vi "Calculate Label Position.vi"(6 "scaling factor":T3={"horizontal"=1.0, "vertical"=1.0} {"vertical" min=0.0; "horizontal" min=0.0}, 8 "layout owner bounds":T4, 9 "scaled object size":T1, 10 "layout object size":T1, 11 "layout label position":T2) -> (3 "scaled label position":T2)   [LabVIEW 2010, in "NI_SE_Front Panel Layout.lvlib"]
uses:
  NI_SE_Front Panel Layout.lvlib
  <vilib>/Utility/miscctls.llb/LVRectTypeDef.ctl
  <vilib>/Utility/miscctls.llb/LVPositionTypeDef.ctl
  XY Scaling Factor.ctl
  <vilib>/Utility/miscctls.llb/LVBoundsTypeDef.ctl
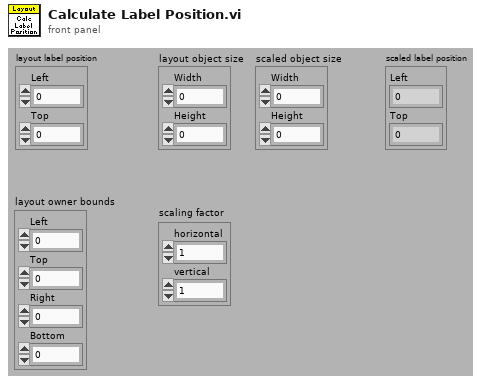
[diagram p1: front panel]
types:
  T1 = typedef "LVBoundsTypeDef.ctl" = cluster{"Width":u32, "Height":u32}
  T2 = typedef "LVPositionTypeDef.ctl" = cluster{"Left":i32, "Top":i32}
  T3 = typedef "NI_SE_Front Panel Layout.lvlib/XY Scaling Factor.ctl" = cluster{"horizontal":dbl, "vertical":dbl}
  T4 = typedef "LVRectTypeDef.ctl" = cluster{"Left":i16, "Top":i16, "Right":i16, "Bottom":i16}
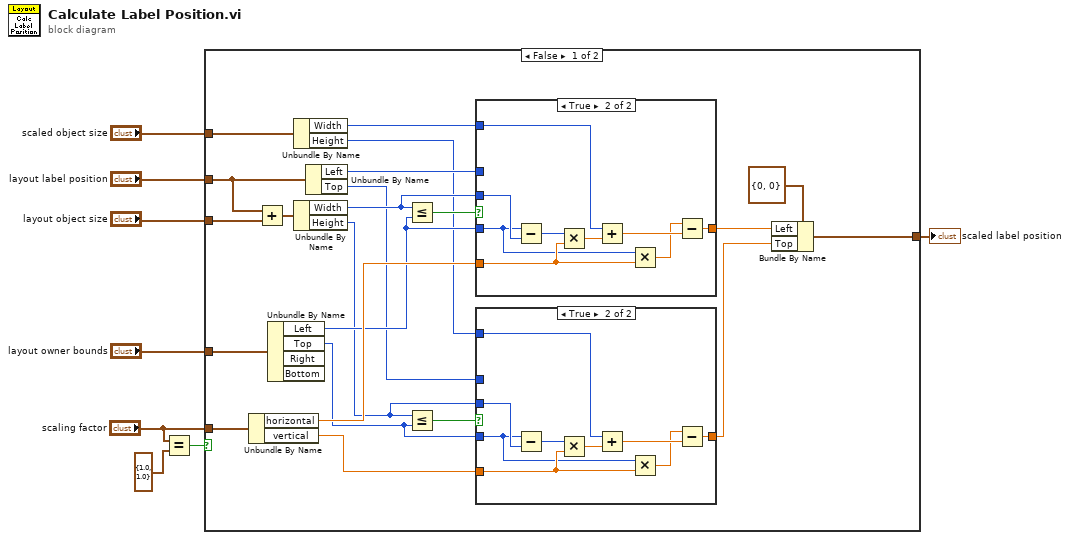
[diagram p0: block diagram]
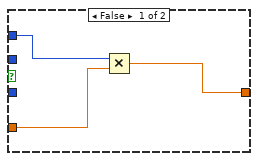
[diagram p2: hidden frame]
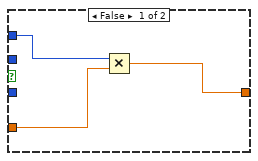
[diagram p3: hidden frame]
diagram:
  n1 = Equal?(x="scaling factor", y=T3 {"horizontal"=1.0, "vertical"=1.0}) -> (x = y?=w2:bool)
  n2 = case shown="False" w2 {
    tunnel: "layout owner bounds" -> [w30 _]
    tunnel: [w27 w55] -> w7
    tunnel: "layout object size" -> [w19 _]
    tunnel: "layout label position" -> [w17 w55]
    tunnel: "scaling factor" -> [w22 _]
    tunnel: "scaled object size" -> [w21 _]
    frame False {
      n3 = Unbundle By Name(w22) -> ("horizontal"=w24:dbl, "vertical"=w13:dbl)
      n4 = Add(x=w17, y=w19) -> (x+y=w18:T1)
      n5 = Unbundle By Name(w30) -> ("Left"=w23:i16, "Top"=w10:i16)  [unwired: 2 out]
      n6 = Unbundle By Name(w21) -> ("Width"=w20:u32, "Height"=w15:u32)
      n7 = Unbundle By Name(w18) -> ("Width"=w25:u32, "Height"=w11:u32)
      n8 = Unbundle By Name(w17) -> ("Left"=w16:i32, "Top"=w14:i32)
      n9 = Less Or Equal?(x=w25, y=w23) -> (x <= y?=w26:bool)
      n10 = Less Or Equal?(x=w11, y=w10) -> (x <= y?=w12:bool)
      n11 = case shown="True" w26 {
        tunnel: [w43 w46] -> w28
        tunnel: w25 -> [_ w54]
        tunnel: w24 -> [w44 w50]
        tunnel: w23 -> [_ w49]
        tunnel: w20 -> [_ w51]
        tunnel: w16 -> [w45 _]
        frame False {
          n12 = Multiply(x=w45, y=w44) -> (x*y=w43:dbl)
        }
        frame True {
          n13 = Subtract(x=w49, y=w54) -> (x-y=w53:u32)
          n14 = Multiply(x=w53, y=w50) -> (x*y=w52:dbl)
          n15 = Add(x=w51, y=w52) -> (x+y=w48:dbl)
          n16 = Multiply(x=w49, y=w50) -> (x*y=w47:dbl)
          n17 = Subtract(x=w47, y=w48) -> (x-y=w46:dbl)
        }
      }
      n18 = case shown="True" w12 {
        tunnel: [w31 w34] -> w9
        tunnel: w11 -> [_ w42]
        tunnel: w13 -> [w32 w38]
        tunnel: w10 -> [_ w37]
        tunnel: w15 -> [_ w39]
        tunnel: w14 -> [w33 _]
        frame False {
          n19 = Multiply(x=w33, y=w32) -> (x*y=w31:dbl)
        }
        frame True {
          n20 = Subtract(x=w37, y=w42) -> (x-y=w41:u32)
          n21 = Multiply(x=w41, y=w38) -> (x*y=w40:dbl)
          n22 = Add(x=w39, y=w40) -> (x+y=w36:dbl)
          n23 = Multiply(x=w37, y=w38) -> (x*y=w35:dbl)
          n24 = Subtract(x=w35, y=w36) -> (x-y=w34:dbl)
        }
      }
      n25 = Bundle By Name(cluster=T2 {"Left"=0, "Top"=0} ("layout label position"), "Left"=w28, "Top"=w9) -> (w27:T2)
    }
    frame True {
    }
  }
  "scaled label position" <- w7
